vi "settings.vi"(6 "Param":string) -> (0 "error out":errorcluster, 2 "Rezult":string)   [LabVIEW 2010]
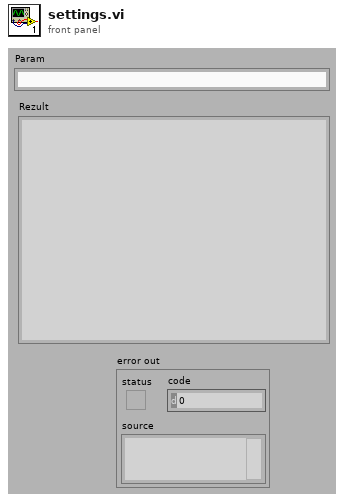
[diagram p1: front panel]
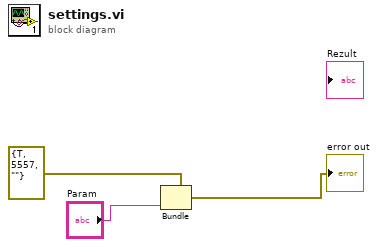
[diagram p0: block diagram]
diagram:
  n1 = Bundle(cluster=errorcluster {"status"=TRUE, "code"=5557, "source"=""} ("error out"), "source"="Param") -> (→"error out":errorcluster)  [unwired: 2 in]
